vi "Execute Tests.vi"(7 "Suite Label":string, 8 "error in (no error)":errorcluster, 11 "Test Runner in":refnum<class "Test Runner.lvclass">) -> (0 "error out":errorcluster, 3 "Test Runner out":refnum<class "Test Runner.lvclass">)   [LabVIEW 2013, in "Caraya.lvlib" / "Test Runner.lvclass"]
uses:
  Test Runner.lvclass
  Test Runner.lvclass/Test Runner.ctl
  Test Suite/Test Suite.lvclass
  Test Suite/Define Test Suite (Default).vi
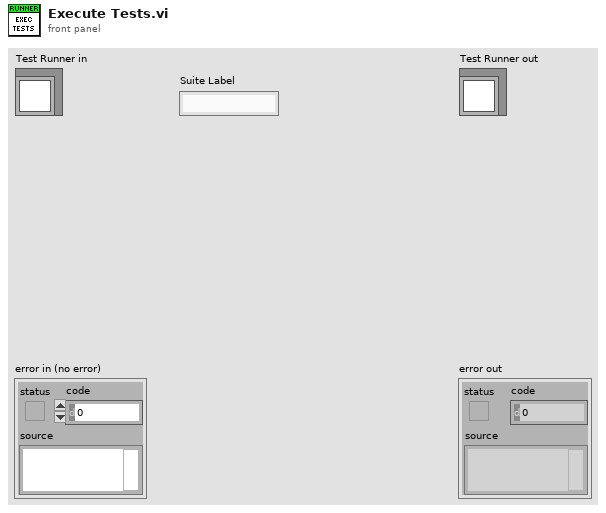
[diagram p1: front panel]
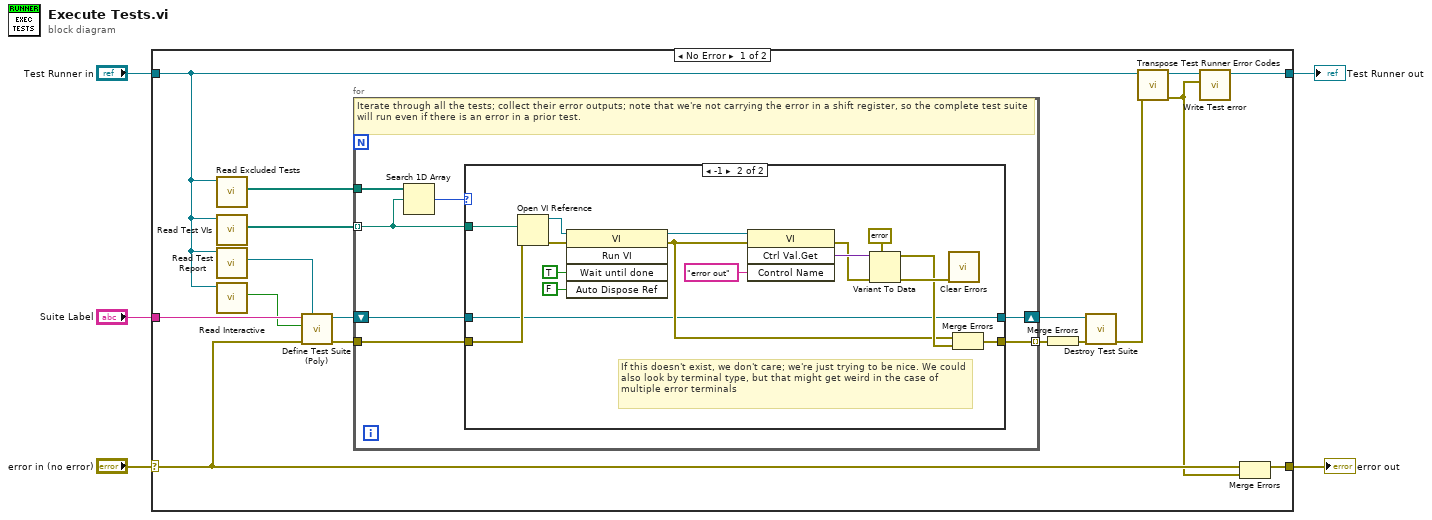
[diagram p0: block diagram]
diagram:
  n1 = case shown="No Error" "error in (no error)" {
    selector: "error in (no error)" -> [w10 w49]
    tunnel: "Suite Label" -> [w22 _]
    tunnel: "Test Runner in" -> [w9 w48]
    tunnel: [w12 w48] -> w3
    tunnel: [w11 w49] -> w2
    frame No Error {
      n2 = call "Read Excluded Tests.vi"("Test Runner in"=w9) -> ("Excluded Tests"=w16:path[])  [unwired: 8 in, 2 out]
      n3 = call-dynamic "Read Test VIs.vi"("Test Runner in"=w9) -> ("Test VIs"=w15:path[])  [unwired: 8 in, 2 out]
      n4 = call "Read Test Report.vi"("Test Runner in"=w9) -> ("Test Report"=w14:refnum<class "Test Report.lvclass">)  [unwired: 8 in, 2 out]
      n5 = call "Read Interactive.vi"("Test Runner in"=w9) -> ("Interactive"=w13:bool)  [unwired: 8 in, 2 out]
      n6 = call-poly "Define Test Suite (Poly).vi"("Test Report (optional)"=w14, "error in (no error)"=w10, "Interactive"=w13, "Label (VI Title)"=w22) -> ("error out"=w20:errorcluster, "Test Suite"=w19:refnum<class "Test Suite.lvclass">)  [unwired: 6 in]
      n7 = for {
        tunnel: w15 -> [w28] mode=indexing
        tunnel: w20 -> [w27]
        tunnel: [w26] -> w21 mode=indexing
        tunnel: w16 -> [w29]
        shift-right: [w23] -> w18
        shift-left: w19 -> [w24]
        # "Iterate through all the tests; collect their error outputs; note that we're not carrying the error in a shift register, so the complete test suite will run even if there is an error in a prior test."
        n8 = Search 1D Array(1D array=w29, element=w28) -> (index of element=w25:i32)  [unwired: 1 in]
        n9 = case shown="-1" w25 {
          tunnel: w28 -> [_ w37]
          tunnel: w27 -> [w31 w36]
          tunnel: [w31 w33] -> w26
          tunnel: w24 -> [w30 w32]
          tunnel: [w30 w32] -> w23
          frame Default {
            # "Test is part of the exclusion list"
          }
          frame -1 {
            # "If this doesn't exist, we don't care; we're just trying to be nice. We could also look by terminal type, but that might get weird in the case of multiple error terminals"
            n10 = Open VI Reference(vi path=w37, error in (no error)=w36) -> (vi reference=w47:refnum<vi>, error out=w46:errorcluster)  [unwired: 4 in]
            n11 = invoke on="Invoke Node" class="VI" method="Run VI"(reference=w47, error in=w46, "Wait until done"=TRUE ("Wait Until Done"), "Auto Dispose Ref"=FALSE ("Auto Dispose Reference")) -> (reference out=w43:refnum<vi>, error out=w34:errorcluster)  [unwired: 1 in, 3 out]
            n12 = invoke on="Invoke Node" class="VI" method="Ctrl Val.Get"(reference=w43, error in=w34, "Control Name"="error out") -> (error out=w40:errorcluster, "Get Control Value Variant"=w41:variant)  [unwired: 1 in, 2 out]
            n13 = Variant To Data(error in=w40, type=errorcluster {"status"=FALSE, "code"=0, "source"=""} ("error out"), Variant=w41) -> (data=w35:errorcluster, error out=w39:errorcluster)
            n14 = call <vilib>:"Clear Errors.vi"("error in (no error)"=w39) -> ()  [unwired: 6 in, 1 out]
            n15 = Merge Errors(w34, w35) -> (w33:errorcluster)
          }
        }
      }
      n16 = Merge Errors(w21) -> (w17:errorcluster)
      n17 = call-dynamic "Destroy Test Suite.vi"("error in (no error)"=w17, "Test Suite in"=w18) -> ("error out"=w7:errorcluster)  [unwired: 9 in]
      n18 = call-dynamic "Transpose Test Runner Error Codes.vi"("error in (no error)"=w7, "Test Runner in"=w9) -> ("error out"=w6:errorcluster, "Test Runner out"=w8:refnum<class "Test Runner.lvclass">)  [unwired: 8 in]
      n19 = call "Write Test error.vi"("Test error"=w6, "Test Runner in"=w8) -> ("Test Runner out"=w12:refnum<class "Test Runner.lvclass">)  [unwired: 8 in, 1 out]
      n20 = Merge Errors(w10, w6) -> (w11:errorcluster)
    }
    frame Error {
    }
  }
  "error out" <- w2
  "Test Runner out" <- w3
